vi "Set Version.vi"(0 "Package Spec":string[](array[string]), 11 "error in (no error)":errorcluster) -> (4 "Build Specification Version":T1, 15 "error out":errorcluster)   [LabVIEW 2021, in "Measurement Builder.lvlib"]
uses:
  Measurement Builder.lvlib
  <vilib>/AppBuilder/AB_API_Simple/Build Specification Version.ctl
  <vilib>/AppBuilder/AB_API_Simple/NI_App_Builder_API.lvlib
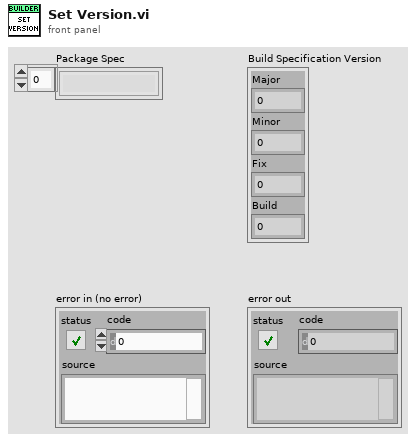
[diagram p1: front panel]
types:
  T1 = typedef "NI_App_Builder_API.lvlib/Build Specification Version.ctl" = cluster{"Major":u16, "Minor":u16, "Fix":u16, "Build":u16}
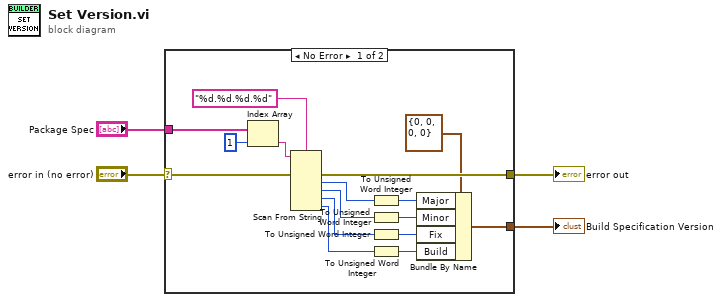
[diagram p0: block diagram]
diagram:
  n1 = case shown="No Error" "error in (no error)" {
    selector: "error in (no error)" -> [w19 w21]
    tunnel: [w20 w21] -> w4
    tunnel: [w10 _] -> w2
    tunnel: "Package Spec" -> [w5 _]
    frame No Error {
      n2 = Index Array(array=w5, index=1) -> (element=w7:string)
      n3 = Scan From String(format string="%d.%d.%d.%d", input string=w7, error in=w19) -> (error out=w20:errorcluster, output 1=w11:i32, output 2=w12:i32, output 3=w13:i32, output 4=w14:i32)  [unwired: 5 in, 2 out]
      n4 = To Unsigned Word Integer(number=w11) -> (unsigned 16bit integer=w15:u16)
      n5 = To Unsigned Word Integer(number=w12) -> (unsigned 16bit integer=w16:u16)
      n6 = To Unsigned Word Integer(number=w13) -> (unsigned 16bit integer=w17:u16)
      n7 = To Unsigned Word Integer(number=w14) -> (unsigned 16bit integer=w18:u16)
      n8 = Bundle By Name(cluster=T1 {"Major"=0, "Minor"=0, "Fix"=0, "Build"=0} ("Build Specification Version"), "Major"=w15, "Minor"=w16, "Fix"=w17, "Build"=w18) -> (w10:T1)
    }
    frame Error {
    }
  }
  "error out" <- w4
  "Build Specification Version" <- w2
